vi "hmi_cheesy_drive.vi"(5 "Quickturn_Sens_Low":dbl=1.2, 7 "Speedturn_Sens_Low":dbl=1.0, 9 "Quick Turn":bool, 10 "Wheel":dbl, 11 "Throttle":dbl) -> (3 "Drive Data":cluster{"Left":dbl, "Right":dbl})   [LabVIEW 2015]
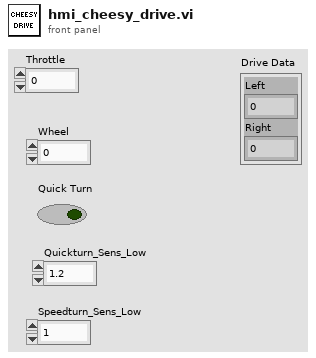
[diagram p1: front panel]
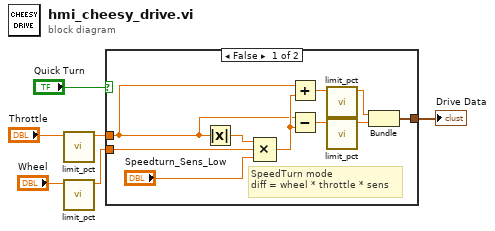
[diagram p0: block diagram]
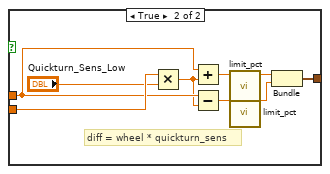
[diagram p2: hidden frame]
diagram:
  n1 = call "limit_pct.vi"("PCT"="Throttle") -> ("PCT Out"=w3:dbl)  [unwired: 10 in]
  n2 = call "limit_pct.vi"("PCT"="Wheel") -> ("PCT Out"=w1:dbl)  [unwired: 10 in]
  n3 = case shown="False" "Quick Turn" {
    tunnel: w1 -> [w16 w25]
    tunnel: w3 -> [w8 w24]
    tunnel: [w14 w22] -> w5
    frame False {
      # "SpeedTurn mode\ndiff = wheel * throttle * sens"
      n4 = Absolute Value(x=w8) -> (abs(x)=w9:dbl)
      n5 = Compound Arithmetic op=MULTIPLY(w9, w16, "Speedturn_Sens_Low") -> (w15:dbl)
      n6 = Add(x=w8, y=w15) -> (x+y=w12:dbl)
      n7 = Subtract(x=w8, y=w15) -> (x-y=w11:dbl)
      n8 = call "limit_pct.vi"("PCT"=w12) -> ("PCT Out"=w13:dbl)  [unwired: 10 in]
      n9 = call "limit_pct.vi"("PCT"=w11) -> ("PCT Out"=w10:dbl)  [unwired: 10 in]
      n10 = Bundle("PCT Out"=w13, "PCT Out"=w10) -> (w14:cluster{"PCT Out":dbl, "PCT Out":dbl})  [unwired: 1 in]
    }
    frame True {
      # "diff = wheel * quickturn_sens"
      n11 = Multiply(x=w25, y="Quickturn_Sens_Low") -> (x*y=w23:dbl)
      n12 = Add(x=w24, y=w23) -> (x+y=w20:dbl)
      n13 = Subtract(x=w24, y=w23) -> (x-y=w18:dbl)
      n14 = call "limit_pct.vi"("PCT"=w20) -> ("PCT Out"=w21:dbl)  [unwired: 10 in]
      n15 = call "limit_pct.vi"("PCT"=w18) -> ("PCT Out"=w19:dbl)  [unwired: 10 in]
      n16 = Bundle("PCT Out"=w21, "PCT Out"=w19) -> (w22:cluster{"PCT Out":dbl, "PCT Out":dbl})  [unwired: 1 in]
    }
  }
  "Drive Data" <- w5
